vi "Material-Automation-LaunchConfigPage.vi"(0 "Configuration Page VI Filepath":path, 5 "Config Dialog Messenger":refnum<class "FTW-Messenger-Actor.lvclass">, 11 "error in":errorcluster) -> (4 "PageID":string, 6 "Initialized?":bool, 8 "Page Messenger":refnum<class "FTW-Messenger-Actor.lvclass">, 15 "error out":errorcluster)   [LabVIEW 2013]
uses:
  Reuse Library/featherweight/Core/Messaging/Messenger.Actor/FTW-Messenger-Actor.lvclass
  Configuration Page Plugin/Material-ConfigPage-Launch.vi
  Configuration Page Plugin/Material-ConfigPage.lvclass
panel:
  # "Inputs"
  # "Outputs"
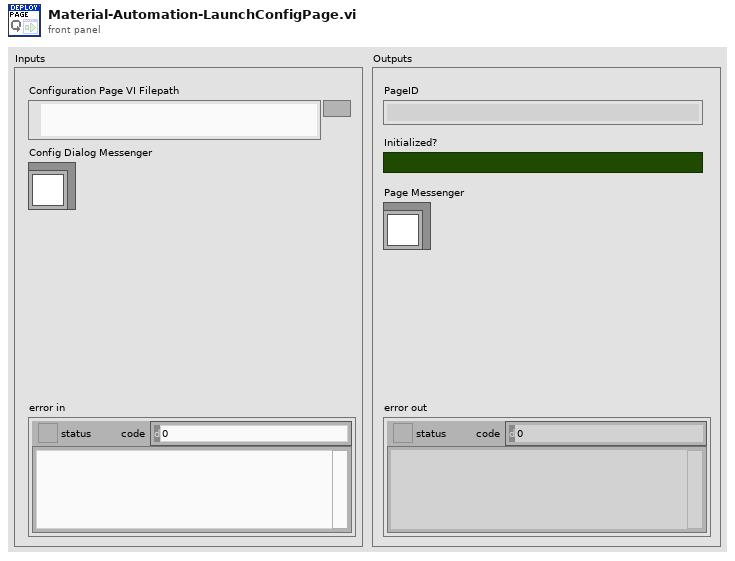
[diagram p1: front panel]
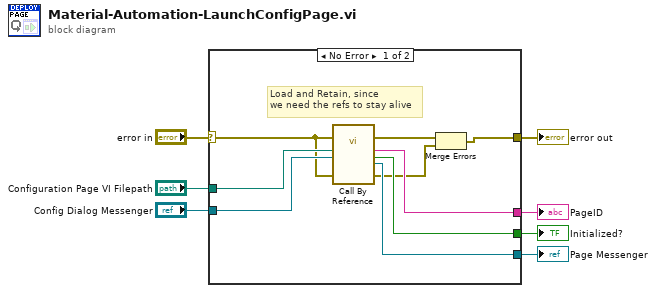
[diagram p0: block diagram]
diagram:
  n1 = case shown="No Error" "error in" {
    selector: "error in" -> [w8 w17]
    tunnel: [w16 w17] -> w7
    tunnel: "Configuration Page VI Filepath" -> [w15 _]
    tunnel: "Config Dialog Messenger" -> [w10 _]
    tunnel: [w12 _] -> w3
    tunnel: [w14 _] -> w2
    tunnel: [w13 _] -> w1
    frame No Error {
      # "Load and Retain, since\nwe need the refs to stay alive"
      n2 = call-by-ref "?"(error in=w8, "Configuration Page VI Filepath"=w15, "Config Dialog Messenger"=w10, "error in"=w8) -> (error out=w9:errorcluster, "PageID"=w14:string, "Initialized?"=w13:bool, "Page Messenger"=w12:refnum<class "FTW-Messenger-Actor.lvclass">, 15:"error out"=w11:errorcluster)  [unwired: 10 in, 1 out]
      n3 = Merge Errors(w9, w11) -> (w16:errorcluster)
    }
    frame Error {
    }
  }
  "error out" <- w7
  "PageID" <- w2
  "Initialized?" <- w1
  "Page Messenger" <- w3
